vi "Working Model.vi"() -> ()   [LabVIEW 2015]
uses:
  <vilib>/addons/JSON API/JSON Value/Set from JSON string.vi
  <vilib>/addons/JSON API/JSON Value/Get Object Item by Name.vi
  <vilib>/addons/JSON API/JSON Scalar/Get as DBL.vi
  <vilib>/imath/engines/lvmath/Plug In/Control Design/BuiltInFunctions/tf/NIMS_CD_tf(STR,Ts).vi
  <vilib>/imathl/engines/lvmath/Functions/Error Handling/Create Error.vi
  <vilib>/imath/engines/lvmath/Plug In/Control Design/BuiltInFunctions/rightdivmx/NIMS_CD_rightdivmx(TF,K).vi
  <vilib>/imath/engines/lvmath/Plug In/Control Design/BuiltInFunctions/powermx/NIMS_CD_powermx(TF,N).vi
  <vilib>/imath/engines/lvmath/Plug In/Control Design/BuiltInFunctions/plus/NIMS_CD_plus(TF,TF).vi
  <vilib>/imath/engines/lvmath/Plug In/Control Design/BuiltInFunctions/plus/NIMS_CD_plus(TF,K).vi
  <vilib>/imath/engines/lvmath/Plug In/Control Design/BuiltInFunctions/rightdivmx/NIMS_CD_rightdivmx(K,TF).vi
  <vilib>/imath/engines/lvmath/Plug In/Control Design/BuiltInFunctions/multmx/NIMS_CD_multmx(K,TF).vi
  <vilib>/imath/engines/lvmath/Functions/Error Handling/MergeErrorsWrapper.vi
  <vilib>/imath/engines/lvmath/Plug In/Control Design/BuiltInFunctions/step/NIMS_CD_[Y,T]=step(TF,[Tinfo]).vi
  <vilib>/imath/engines/lvmath2/RunTimeEngine/NodeEndStatement/NIMS_NodeEndStatement_Output.vi
  <instcachedir>/0/NIMS_NodeEndStatement_Output_53EC0D466D134D7ABD903AC30B43404B.lvgen/NIMS_NodeEndStatement_Output_53EC0D466D134D7ABD903AC30B43404B_001.vi
  <vilib>/imath/engines/lvmath2/RunTimeEngine/ErrorHandling/NIMS_Finalize Error.vi
  <vilib>/addons/JSON API/JSON Value/JSON Value.lvclass
  <vilib>/addons/JSON API/Get Polymorphic/JSON GetSet.lvlib
  <vilib>/addons/JSON API/JSON Scalar/JSON Scalar.lvclass
panel:
  in  "stop":bool
  out "r1":dbl
  out "R":dbl
  out "C":dbl
  out "L":dbl
  out "D":dbl
  out "Vin":dbl
  out "F":dbl
  out "data in":string="Hello World!"
  out "error out":errorcluster
  out "In":string
  out "Processed":string
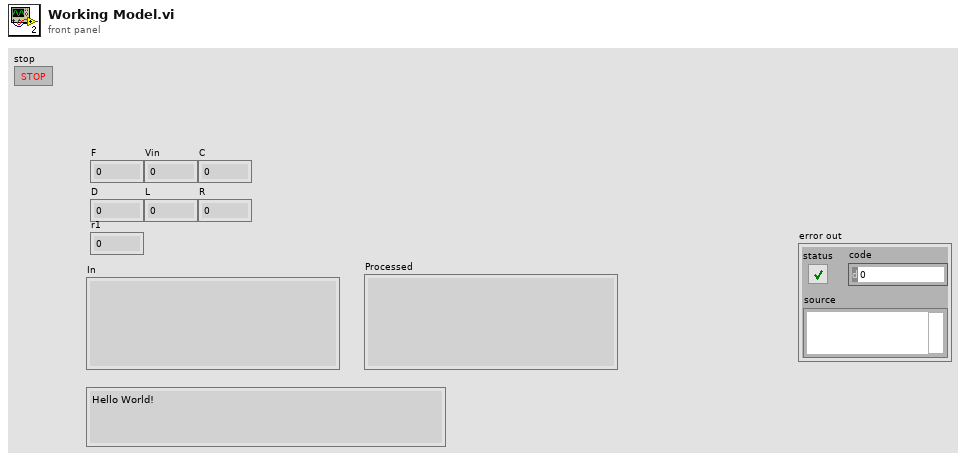
[diagram p1: front panel]
types:
  T1 = cluster{"Vo":dbl, "Io":dbl, "P":dbl, "deltaIL":dbl}
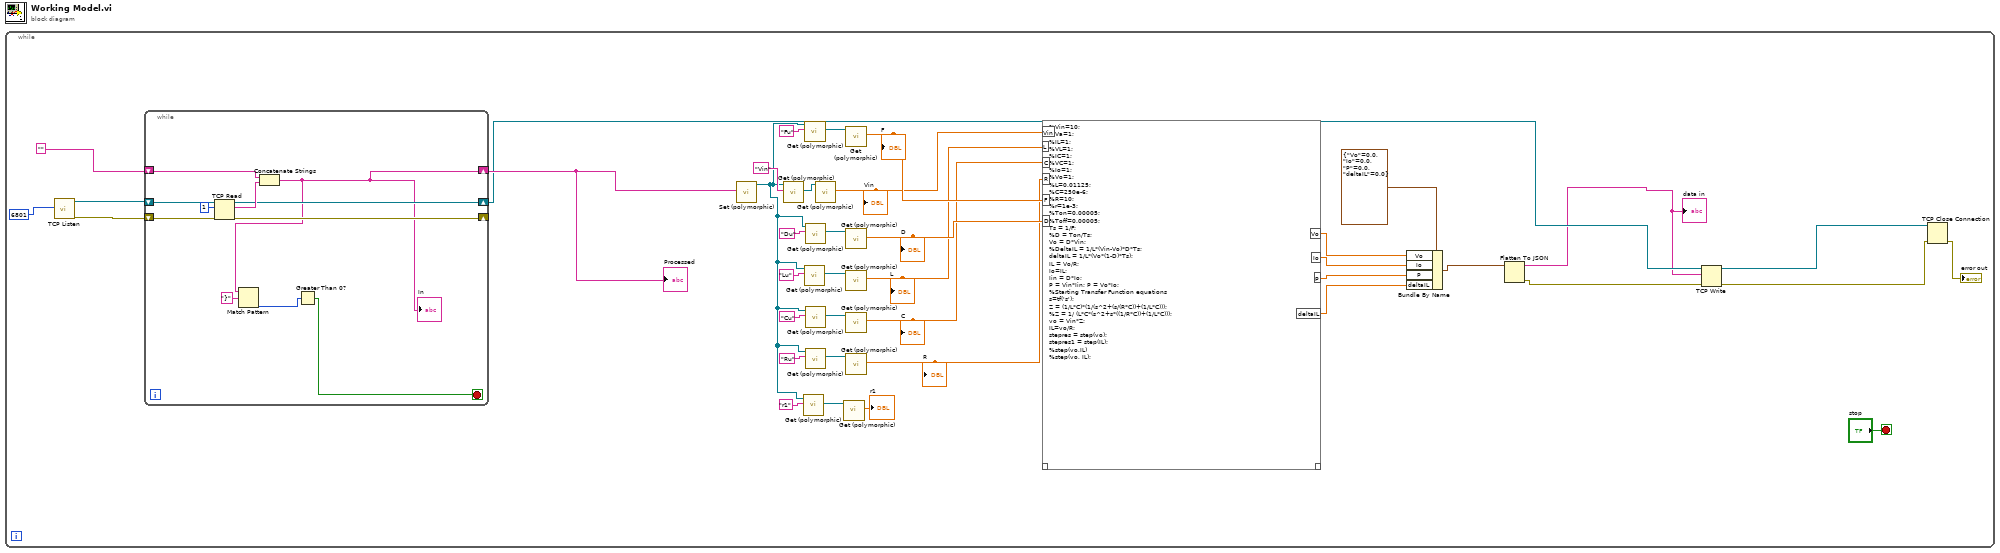
[diagram p0: block diagram]
diagram:
  n1 = while {
    stop <- "stop" stop-if-true
    n2 = call <vilib>:"TCP Listen.vi"("port"=u16 6801) -> ("error out"=w38:errorcluster, "connection ID"=w37:refnum<k5>)  [unwired: 6 in, 3 out]
    n3 = while {
      shift-right: [w44] -> w24
      shift-left: "" -> [w51]
      shift-right: [w48] -> _
      shift-left: w38 -> [w50]
      shift-right: [w45] -> w14
      shift-left: w37 -> [w49]
      stop <- w41 stop-if-true
      n4 = TCP Read(connection ID=w49, bytes to read=1, error in (no error)=w50) -> (connection ID out=w45:refnum<k5>, data out=w46:string, error out=w48:errorcluster)  [unwired: 2 in]
      n5 = Concatenate Strings(w51, w46) -> (w44:string)
      "In" <- w44
      n6 = Match Pattern(string=w44, regular expression="}") -> (offset past match=w42:i32)  [unwired: 1 in, 3 out]
      n7 = Greater Than 0?(x=w42) -> (x > 0?=w41:bool)
    }
    "Processed" <- w24
    n8 = call-poly <vilib>:"Set (polymorphic).vi"("JSON stream"=w24) -> ("JSON Value out"=w4:refnum<class "JSON Value.lvclass">)  [unwired: 8 in, 2 out]
    n9 = call-poly <vilib>:"Get (polymorphic).vi"("name"="Vin", "JSON Value In"=w4) -> ("Value"=w35:refnum<class "JSON Value.lvclass">)  [unwired: 6 in, 3 out]
    n10 = call-poly <vilib>:"Get (polymorphic).vi"("name"="r1", "JSON Value In"=w4) -> ("Value"=w6:refnum<class "JSON Value.lvclass">)  [unwired: 6 in, 3 out]
    n11 = call-poly <vilib>:"Get (polymorphic).vi"("name"="Lu", "JSON Value In"=w4) -> ("Value"=w32:refnum<class "JSON Value.lvclass">)  [unwired: 6 in, 3 out]
    n12 = call-poly <vilib>:"Get (polymorphic).vi"("name"="Fu", "JSON Value In"=w4) -> ("Value"=w26:refnum<class "JSON Value.lvclass">)  [unwired: 6 in, 3 out]
    n13 = call-poly <vilib>:"Get (polymorphic).vi"("name"="Du", "JSON Value In"=w4) -> ("Value"=w34:refnum<class "JSON Value.lvclass">)  [unwired: 6 in, 3 out]
    n14 = call-poly <vilib>:"Get (polymorphic).vi"("name"="Cu", "JSON Value In"=w4) -> ("Value"=w30:refnum<class "JSON Value.lvclass">)  [unwired: 6 in, 3 out]
    n15 = call-poly <vilib>:"Get (polymorphic).vi"("name"="Ru", "JSON Value In"=w4) -> ("Value"=w28:refnum<class "JSON Value.lvclass">)  [unwired: 6 in, 3 out]
    n16 = call-poly <vilib>:"Get (polymorphic).vi"("JSON Value in"=w35) -> ("Number"=w22:dbl)  [unwired: 8 in, 2 out]
    "Vin" <- w22
    n17 = call-poly <vilib>:"Get (polymorphic).vi"("JSON Value in"=w6) -> ("Number"=→"r1":dbl)  [unwired: 8 in, 2 out]
    n18 = call-poly <vilib>:"Get (polymorphic).vi"("JSON Value in"=w26) -> ("Number"=w23:dbl)  [unwired: 8 in, 2 out]
    "F" <- w23
    n19 = call-poly <vilib>:"Get (polymorphic).vi"("JSON Value in"=w34) -> ("Number"=w21:dbl)  [unwired: 8 in, 2 out]
    "D" <- w21
    n20 = call-poly <vilib>:"Get (polymorphic).vi"("JSON Value in"=w32) -> ("Number"=w20:dbl)  [unwired: 8 in, 2 out]
    "L" <- w20
    n21 = call-poly <vilib>:"Get (polymorphic).vi"("JSON Value in"=w30) -> ("Number"=w19:dbl)  [unwired: 8 in, 2 out]
    "C" <- w19
    n22 = call-poly <vilib>:"Get (polymorphic).vi"("JSON Value in"=w28) -> ("Number"=w18:dbl)  [unwired: 8 in, 2 out]
    "R" <- w18
    n23 = mathscript code="%Vin=10;\n%Va=1;\n%IL=1;\n%VL=1;\n%IC=1;\n%VC=1;\n%Io=1;\n%Vo=1;\n%L=0.01125;\n%C=250e-6;\n%R=10;\n%r=1e-3;\n%Ton=0.00005;\n%Toff=0.00005;\nTs = 1/F;\n%D = Ton/Ts;\nVo = D*Vin;\n%DeltaIL = 1/L*(Vin-Vo)*D*Ts;\ndeltaIL = 1/L*(Vo*(1-D)*Ts);\nIL = Vo/R;\nIo=IL;\nIin = D*Io;\nP = Vin*Iin; P = Vo*Io;\n%Starting Transfer Function equations\ns=tf('s');\nZ = (1/L*C)*(1/(s^2+(s/(R*C))+(1/L*C)));\n%Z = 1/ (L*C*(s^2+s*((1/R*C))+(1/L*C)));\nvo = Vin*Z;\nIL=vo/R;\nstepres = step(vo);\nstepres1 = step(IL);\n%step(vo,IL)\n%step(vo, IL);"("Vin"=w22, "L"=w20, "C"=w19, "R"=w18, "F"=w23, "D"=w21) -> ("Vo"=w12:dbl, "Io"=w11:dbl, "P"=w10:dbl, "deltaIL"=w9:dbl)  [unwired: 1 in, 1 out]
    n24 = Bundle By Name(cluster=T1 {"Vo"=0.0, "Io"=0.0, "P"=0.0, "deltaIL"=0.0} ("input cluster"), "Vo"=w12, "Io"=w11, "P"=w10, "deltaIL"=w9) -> (w8:T1)
    n25 = Flatten To JSON(anything=w8) -> (JSON string=w7:string, 11:w2:errorcluster)  [unwired: 2 in]
    "data in" <- w7
    n26 = TCP Write(connection ID=w14, data in=w7, error in (no error)=w2) -> (connection ID out=w17:refnum<k5>, error out=w16:errorcluster)  [unwired: 1 in, 1 out]
    n27 = TCP Close Connection(connection ID=w17, error in (no error)=w16) -> (error out=→"error out":errorcluster)  [unwired: 1 in, 1 out]
  }
